vi "reflectiesensor_lezen (SubVI).vi"(8 "error in (no error)":errorcluster, 11 "namen van analoge inputs  in":tag[](array[tag])) -> (0 "error out":errorcluster, 3 "Values":dbl[](array[numeric]))   [LabVIEW 2019]
uses:
  <vilib>/myRIO/Instrument Drivers/Onboard IO/AI/AI.lvlib
  <vilib>/myRIO/Express VI/Onboard IO/AI/AI Express VI.xnode
  <vilib>/myRIO/Common/Instrument Driver Framework/Utilities/typedefs/Analog Scaling Constants.ctl
  <vilib>/myRIO/Common/Instrument Driver Framework/Utilities/typedefs/Analog Scaling Constants List.ctl
  <vilib>/myRIO/Common/Instrument Driver Framework/myRIO v1.0/AI/typedefs/AI Channels Enum.ctl
  <vilib>/myRIO/Common/Instrument Driver Framework/myRIO v1.0/AI/typedefs/AI Channels List.ctl
  <vilib>/myRIO/Common/Instrument Driver Framework/Utilities/typedefs/Generic FPGA Reference.ctl
  <vilib>/myRIO/Common/Instrument Driver Framework/Utilities/typedefs/myRIO v1.0 Reference.ctl
  <vilib>/myRIO/Common/Instrument Driver Framework/Utilities/typedefs/Hardware Version Enum.ctl
  <vilib>/myRIO/Common/Instrument Driver Framework/Utilities/typedefs/myRIO Generic Hardware Reference.ctl
  <vilib>/myRIO/Instrument Drivers/Onboard IO/AI/typedefs/AI Reference.ctl
  <vilib>/myRIO/Instrument Drivers/Onboard IO/AI/vis/myRIO AI Open.xnode
  <vilib>/myRIO/Common/Instrument Driver Framework/Utilities/vis/Is FPGA Ref Available.vi
  <vilib>/myRIO/Common/Instrument Driver Framework/myRIO v1.0/AI/vis/myRIO v1.1 Open AI.vi
  <vilib>/userDefined/High Color/nirio_resource_hc.ctl
panel:
  out "B/AI2 (Pin 7)":dbl
  out "B/AI1 (Pin 5)":dbl
  out "B/AI0 (Pin 3)":dbl
  out "A/AI2 (Pin 7)":dbl
  out "A/AI1 (Pin 5)":dbl
  out "A/AI0 (Pin 3)":dbl
  in  "stop":bool
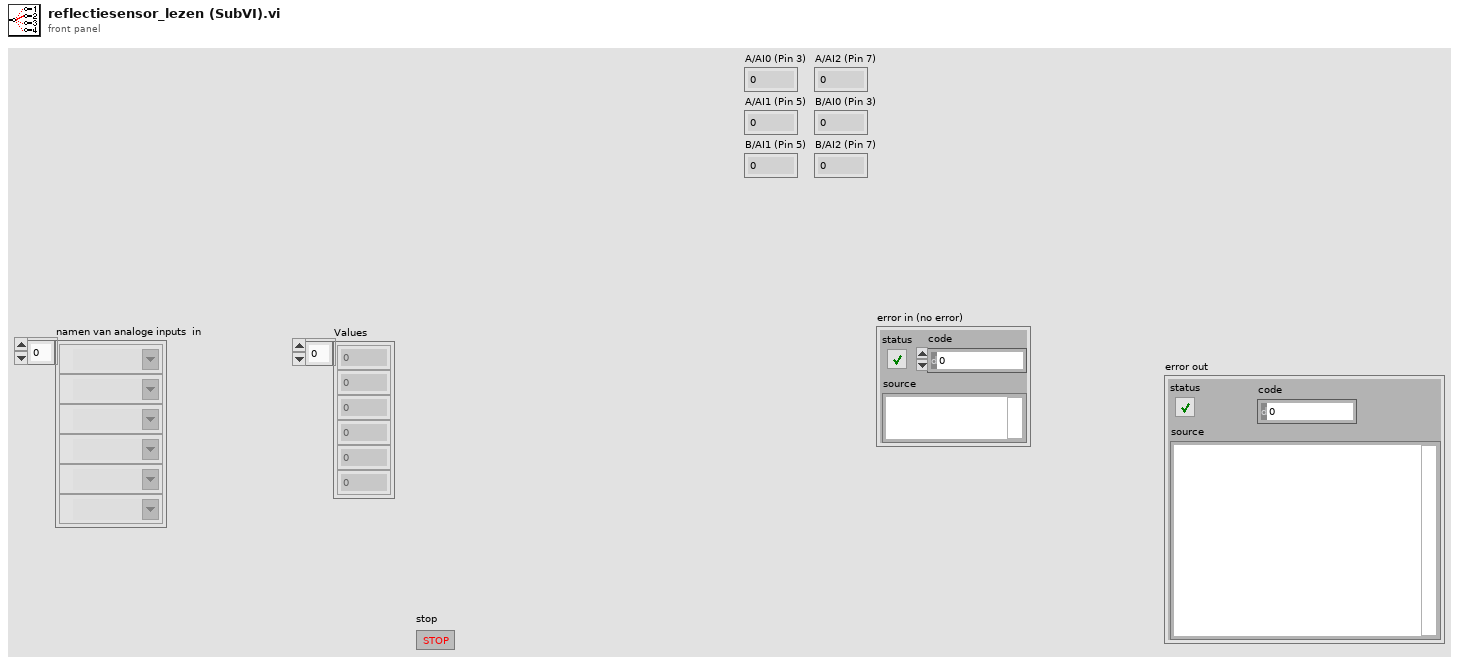
[diagram p1: front panel]
types:
  T1 = typedef "AI.lvlib/AI Reference.ctl" = cluster{"myRIO Reference":T2, "AI Channels List":T6, "AI Scaling Constants List":T8}
  T2 = typedef "myRIO Generic Hardware Reference.ctl" = cluster{"myRIO Model":T3, "myRIO Hardware Reference":T4}
  T3 = typedef "Hardware Version Enum.ctl" = enum16{"Unknown", "myRIO-1900", "myRIO-1950", "roboRIO", "NI ELVIS RIO CM", "ELVIS III"}
  T4 = typedef "myRIO v1.0 Reference.ctl" = cluster{"Generic FPGA Reference":T5, "Allow multiple opens":bool}
  T5 = typedef "Generic FPGA Reference.ctl" = refnum<k20>
  T6 = typedef "AI Channels List.ctl" = T7[]
  T7 = typedef "AI Channels Enum.ctl" = enum16{"Not Connected", "AudioIn/Left", "AudioIn/Right", "C/AI0", "C/AI1", "A/AI0", "A/AI1", "A/AI2", "A/AI3", "A/AI4", "A/AI5", "A/AI6", "A/AI7", "B/AI0", "B/AI1", "B/AI2", "B/AI3", "B/AI4", "B/AI5", "B/AI6", "B/AI7", "AI/AI0", "AI/AI1", "AI/AI2", "AI/AI3", "A/AI0 (DIFF)", "A/AI1 (DIFF)", "A/AI2 (DIFF)", "A/AI3 (DIFF)", "B/AI0 (DIFF)", "B/AI1 (DIFF)", "B/AI2 (DIFF)", "B/AI3 (DIFF)"}
  T8 = typedef "Analog Scaling Constants List.ctl" = T9[]
  T9 = typedef "Analog Scaling Constants.ctl" = cluster{"LSB Weight (Volts)":dbl, "Offset (Volts)":dbl, "Signed?":bool}
  T10 = typedef "nirio_resource_hc.ctl" = tag
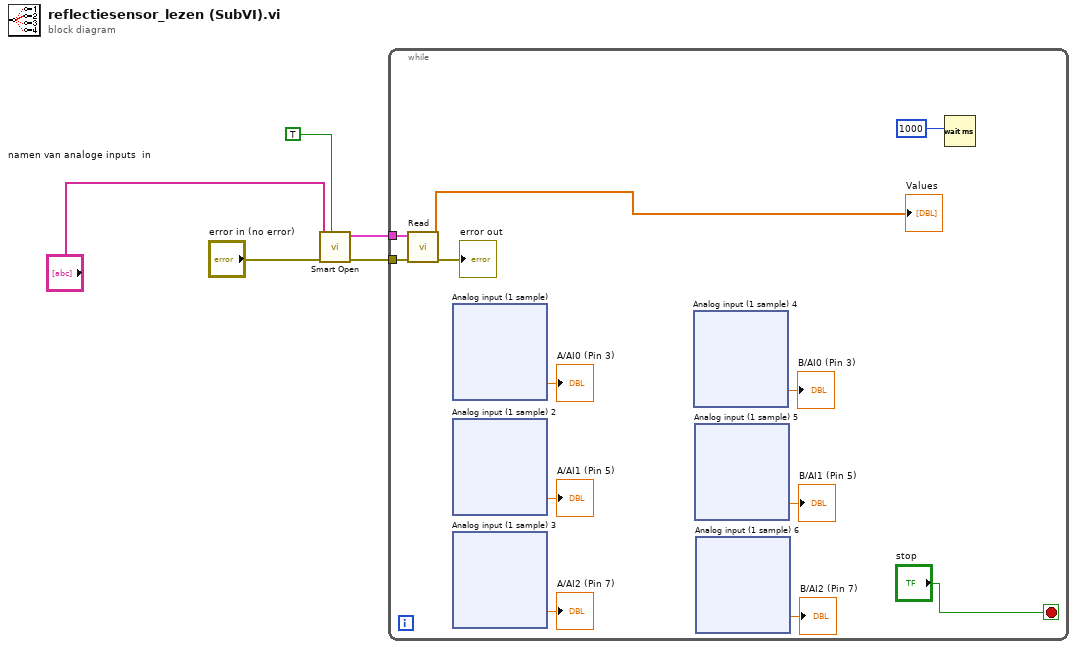
[diagram p0: block diagram]
diagram:
  n1 = call <vilib>:"Smart Open.vi"("Allow multiple opens?"=TRUE, "error in (no error)"="error in (no error)", "Channel Names"="namen van analoge inputs  in") -> ("error out"=w2:errorcluster, "AI Ref Out"=w3:T1)  [unwired: 7 in]
  n2 = while {
    tunnel: w3 -> [w17]
    tunnel: w2 -> [w16]
    stop <- "stop" stop-if-true
    n3 = call <vilib>:"Read.vi"("error in (no error)"=w16, "AI Ref In"=w17) -> ("error out"=→"error out":errorcluster, "Values"=→"Values":dbl[])  [unwired: 7 in, 1 out]
    n4 = xnode "Analog input (1 sample)"() -> ("A/AI0 (Pin 3)"=→"A/AI0 (Pin 3)":dbl)  [unwired: 1 in, 1 out]
    n5 = xnode "Analog input (1 sample) 2"() -> ("A/AI1 (Pin 5)"=→"A/AI1 (Pin 5)":dbl)  [unwired: 1 in, 1 out]
    n6 = xnode "Analog input (1 sample) 3"() -> ("A/AI2 (Pin 7)"=→"A/AI2 (Pin 7)":dbl)  [unwired: 1 in, 1 out]
    n7 = xnode "Analog input (1 sample) 4"() -> ("B/AI0 (Pin 3)"=→"B/AI0 (Pin 3)":dbl)  [unwired: 1 in, 1 out]
    n8 = xnode "Analog input (1 sample) 5"() -> ("B/AI1 (Pin 5)"=→"B/AI1 (Pin 5)":dbl)  [unwired: 1 in, 1 out]
    n9 = xnode "Analog input (1 sample) 6"() -> ("B/AI2 (Pin 7)"=→"B/AI2 (Pin 7)":dbl)  [unwired: 1 in, 1 out]
    n10 = Wait (ms)(milliseconds to wait=1000) -> ()  [unwired: 1 out]
  }
